vi "RotationMatrixBetweenPlanes.vi"(8 "error in":errorcluster, 9 "Plane 2 Coefficients":T1, 11 "Plane 1 Coefficients":T1) -> (0 "error out":errorcluster, 3 "Rotation Matrix":T2)   [LabVIEW 2020, in "ar.lvlib"]
uses:
  ar.lvlib
  Plane Coefficients.ctl
  <vilib>/Analysis/Matrix/Datatypes/RealMatrix.ctl
  <vilib>/Analysis/baseanly.llb/Real Dot Product.vi
  <vilib>/Analysis/7linalg.llb/Real Matrix Power.vi
  <vilib>/Analysis/_algsub.llb/Real Matrix Norm.vi
  <vilib>/Analysis/7linalg.llb/Create Special Real Matrix.vi
  <vilib>/Analysis/Matrix/NI_Matrix.lvlib
  <vilib>/Analysis/NI_AALPro.lvlib
  <vilib>/Analysis/NI_AALBase.lvlib
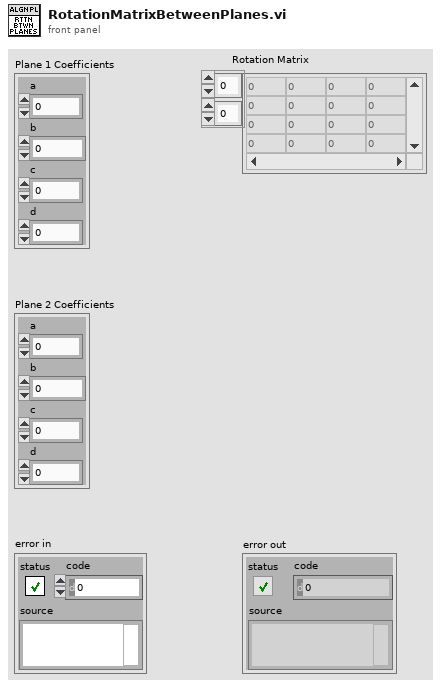
[diagram p1: front panel]
types:
  T1 = typedef "ar.lvlib/Plane Coefficients.ctl" = cluster{"a":dbl, "b":dbl, "c":dbl, "d":dbl}
  T2 = typedef "NI_Matrix.lvlib/RealMatrix.ctl" = dbl[][]
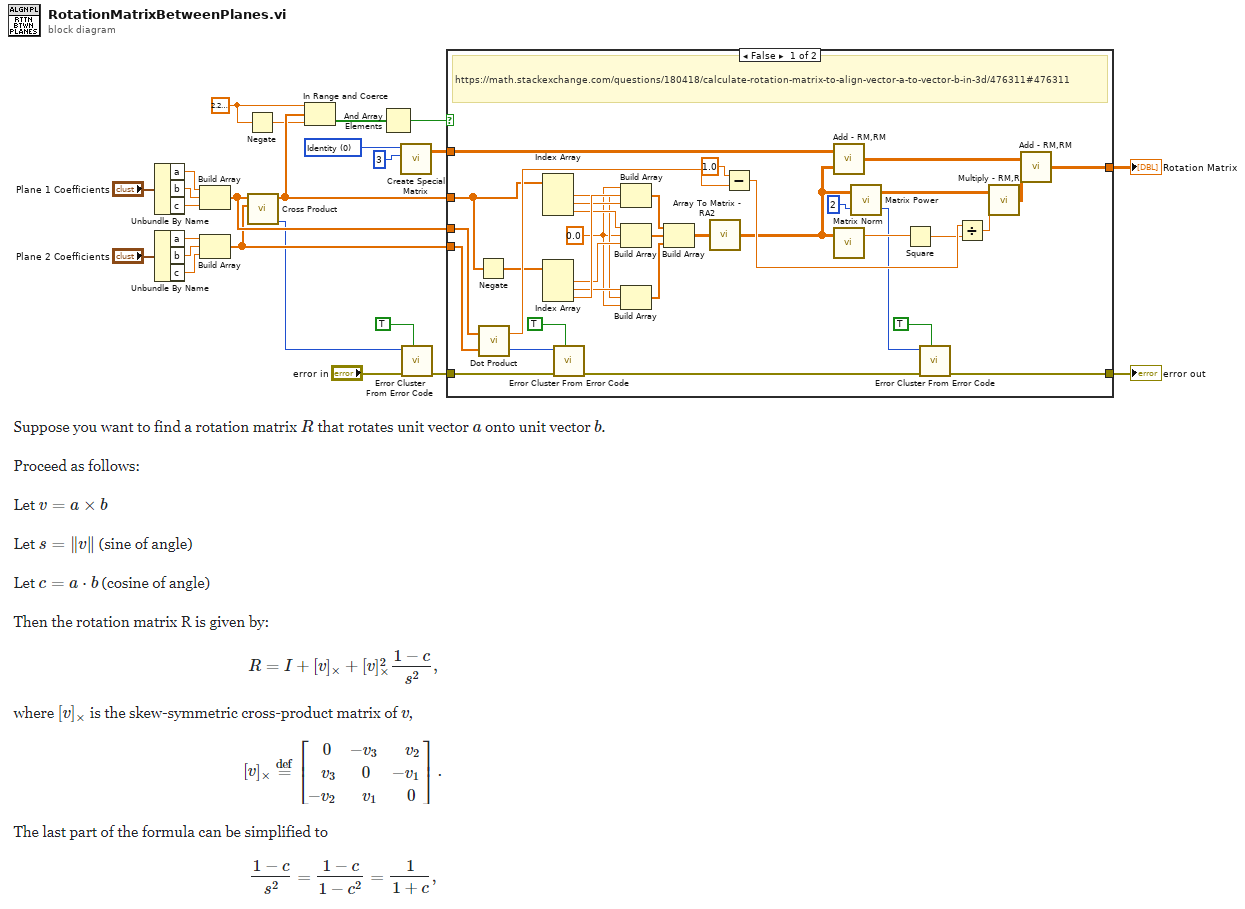
[diagram p0: block diagram]
diagram:
  w14 = 2.220446049250313e-16
  w24 = 0 items=["Identity", "Diagonal", "Toeplitz", "Vandermonde", "Companion", "Hankel", "Hadamard", "Wilkinson", "Hilbert", "Inverse Hilbert", "Rosser", "Pascal"] ("matrix type")
  n1 = Unbundle By Name("Plane 1 Coefficients") -> ("a"=w21:dbl, "b"=w20:dbl, "c"=w19:dbl)
  n2 = Unbundle By Name("Plane 2 Coefficients") -> ("a"=w9:dbl, "b"=w8:dbl, "c"=w7:dbl)
  n3 = Build Array(w21, w20, w19) -> (w18:dbl[])
  n4 = Build Array(w9, w8, w7) -> (w6:dbl[])
  n5 = Negate(x=w14) -> (-x=w13:dbl)
  n6 = call <vilib>:"Cross Product.vi"("B Vector"=w6, "A Vector"=w18) -> ("error"=w5:i32, "Cross Product"=w15:dbl[])  [unwired: 8 in]
  n7 = In Range and Coerce(upper limit=w14, x=w15, lower limit=w13) -> (In Range?=w12:bool[])  [unwired: 1 out]
  n8 = And Array Elements(Boolean array=w12) -> (logical AND=w11:bool)
  n9 = call-poly <vilib>:"Create Special Matrix.vi"("matrix type"=w24, "matrix size"=3) -> ("Special Matrix"=w22:T2)  [unwired: 3 in, 1 out]
  n10 = call <vilib>:"Error Cluster From Error Code.vi"("show call chain? (False)"=TRUE, "error in (no error)"="error in", "error code (0)"=w5) -> ("error out"=w4:errorcluster)  [unwired: 6 in]
  n11 = case shown="False" w11 {
    tunnel: w22 -> [w58 w61]
    tunnel: w18 -> [w47 _]
    tunnel: w6 -> [w46 _]
    tunnel: [w33 w61] -> w16
    tunnel: w15 -> [w32 _]
    tunnel: w4 -> [w29 w60]
    tunnel: [w27 w60] -> w2
    frame False {
      w38 = 0.0 ("element")
      # "https://math.stackexchange.com/questions/180418/calculate-rotation-matrix-to-align-vector-a-to-vector-b-in-3d/476311#476311"
      n12 = Negate(x=w32) -> (-x=w45:dbl[])
      n13 = call-poly <vilib>:"Dot Product.vi"("Y Vector"=w46, "X Vector"=w47) -> ("error"=w31:i32, "X * Y"=w56:dbl)
      n14 = Index Array(array=w32) -> (element #1=w39:dbl, element #2=w43:dbl, element #3=w42:dbl)  [unwired: 3 in]
      n15 = Index Array(array=w45) -> (element #1=w41:dbl, element #2=w40:dbl, element #3=w44:dbl)  [unwired: 3 in]
      n16 = call <vilib>:"Error Cluster From Error Code.vi"("show call chain? (False)"=TRUE, "error in (no error)"=w29, "error code (0)"=w31) -> ("error out"=w28:errorcluster)  [unwired: 6 in]
      n17 = Build Array(w38, w44, w43) -> (w35:dbl[])
      n18 = Build Array(w42, w38, w41) -> (w36:dbl[])
      n19 = Build Array(w40, w39, w38) -> (w37:dbl[])
      n20 = Build Array(w35, w36, w37) -> (w34:dbl[][])
      n21 = call <vilib>:"Array To Matrix - RA2.vi"("Real 2D Array"=w34) -> ("Real Matrix"=w53:T2)
      n22 = Subtract(x=1.0, y=w56) -> (x-y=w55:dbl)
      n23 = call <vilib>:"Add - RM,RM.vi"("Real Matrix B"=w53, "Real Matrix A"=w58) -> ("A + B"=w52:T2)
      n24 = call-poly <vilib>:"Matrix Norm.vi"("Input Matrix"=w53) -> ("norm"=w50:dbl)  [unwired: 1 in, 1 out]
      n25 = call-poly <vilib>:"Matrix Power.vi"("n"=2, "Input Matrix"=w53) -> ("error"=w30:i32, "Matrix Power"=w54:T2)
      n26 = Square(x=w50) -> (x^2=w49:dbl)
      n27 = call <vilib>:"Error Cluster From Error Code.vi"("show call chain? (False)"=TRUE, "error in (no error)"=w28, "error code (0)"=w30) -> ("error out"=w27:errorcluster)  [unwired: 6 in]
      n28 = Divide(x=w55, y=w49) -> (x/y=w48:dbl)
      n29 = call <vilib>:"Multiply - RM,R.vi"("Real Scalar c"=w48, "Real Matrix A"=w54) -> ("A * c"=w51:T2)
      n30 = call <vilib>:"Add - RM,RM.vi"("Real Matrix B"=w51, "Real Matrix A"=w52) -> ("A + B"=w33:T2)
    }
    frame True {
      # "Planes Already Aligned"
    }
  }
  "Rotation Matrix" <- w16
  "error out" <- w2
